vi "Call Vaa3D.vi"(8 "error in (no error)":errorcluster, 9 "spacing_between_points":dbl, 10 "Call_Vaa3D":bool, 11 "Z-stack folder path":path) -> (0 "error out":errorcluster)   [LabVIEW 2017]
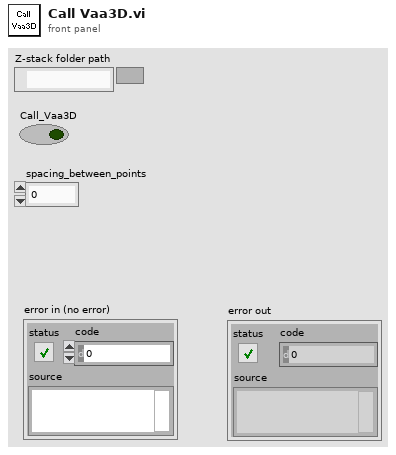
[diagram p1: front panel]
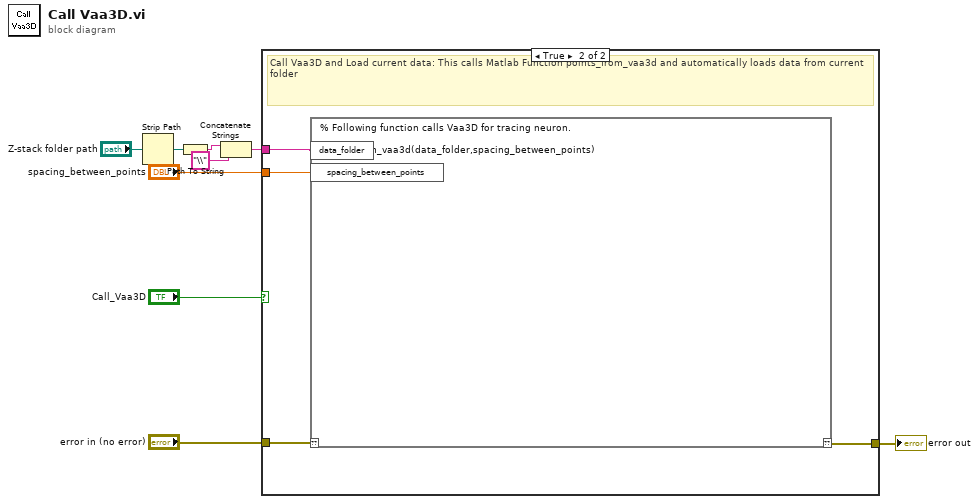
[diagram p0: block diagram]
diagram:
  n1 = Strip Path(path="Z-stack folder path") -> (stripped path=w3:path)  [unwired: 1 out]
  n2 = Path To String(path=w3) -> (string=w4:string)
  n3 = Concatenate Strings(w4, "\\" ("string")) -> (w2:string)
  n4 = case shown="True" "Call_Vaa3D" {
    tunnel: "spacing_between_points" -> [_ w14]
    tunnel: w2 -> [_ w11]
    tunnel: [w10 w13] -> w6
    tunnel: "error in (no error)" -> [w10 w12]
    frame False {
    }
    frame True {
      # "Call Vaa3D and Load current data: This calls Matlab Function points_from_vaa3d and automatically loads data from current folder"
      n5 = script code="% Following function calls Vaa3D for tracing neuron.\n\npoints_from_vaa3d(data_folder,spacing_between_points)"("??"=w12, "spacing_between_points"=w14, "data_folder"=w11) -> ("??"=w13:errorcluster)
    }
  }
  "error out" <- w6
